vi "DSF.UDP.Configuration.Plugin.Create.vi"(6 "Cycle Timing Factors":T1={"Decimation"=1, "Offset"=0}, 8 "error in (no error)":errorcluster, 10 "Name":string, 11 "UDP Transfer Group Configurations":refnum<class "DSF.UDP.Configuration.Transfer Group.lvclass">[](array[class])) -> (0 "error out":errorcluster, 3 "UDP Plugin Configuration out":refnum<class "DSF.UDP.Configuration.Plugin.lvclass">)   [LabVIEW 2016, in "DSF.UDP.Configuration.Plugin.lvclass"]
uses:
  DSF.UDP.Configuration.Plugin.lvclass
  C:/Git/SourceTree/DSF/Source/Shared/Classes/Plugin/DSF.Shared.Configuration.Plugin.lvclass
  DSF.UDP.Configuration.Transfer Group.lvclass
  C:/Git/SourceTree/DSF/Source/Shared/Classes/Transfer Group/DSF.Shared.Configuration.Transfer Group.lvclass
  Source/Shared/Typedefs/DSF.Shared.Typedefs.Cycle Timing Factors.ctl
  Source/Shared/Classes/Plugin/DSF.Shared.Configuration.Plugin.lvclass
  Source/DSF.Shared.lvlib
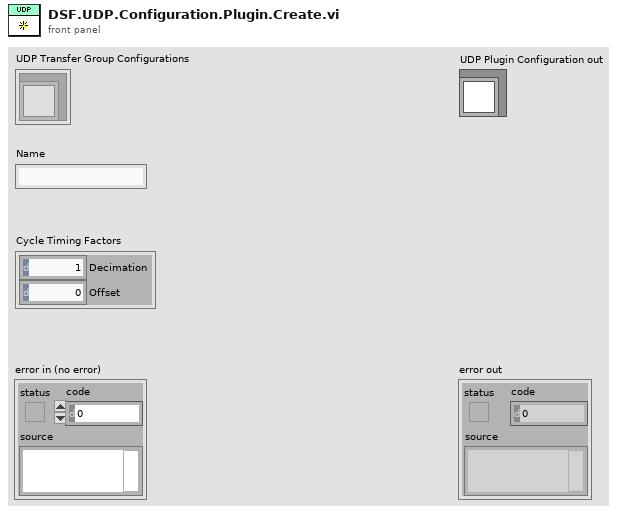
[diagram p1: front panel]
types:
  T1 = typedef "DSF.Shared.lvlib/DSF.Shared.Typedefs.Cycle Timing Factors.ctl" = cluster{"Decimation":u64, "Offset":u64}
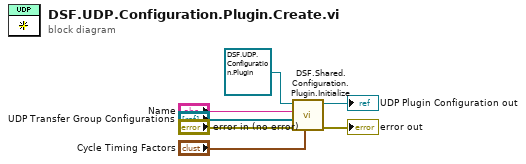
[diagram p0: block diagram]
diagram:
  n1 = call "DSF.Shared.Configuration.Plugin.Initialize.vi"("Cycle Timing Factors"="Cycle Timing Factors", "error in (no error)"="error in (no error)", "Transfer Group Configurations"="UDP Transfer Group Configurations", "Name"="Name", "Plugin Configuration in"=refnum<class "DSF.UDP.Configuration.Plugin.lvclass"> refnum ("UDP Plugin Configuration in")) -> ("error out"=→"error out":errorcluster, "Plugin Configuration out"=→"UDP Plugin Configuration out":refnum<class "DSF.UDP.Configuration.Plugin.lvclass">)  [unwired: 5 in]
